vi "Post Destroy.vi"(8 "Error in":errorcluster, 10 "Actor":refnum<class "Actor.lvclass">) -> ()   [LabVIEW 2020, in "jettl.lvlib" / "Actor.lvlib"]
uses:
  Actor.lvlib
  Actor/Actor.lvclass
  Attributes/Attributes/Attributes.lvclass
  Has Destroyed Msg/Has Destroyed Msg.lvlib
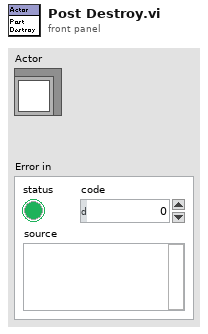
[diagram p1: front panel]
types:
  T1 = typedef "jettl.lvlib/Actor.lvlib/Created Aliases.ctl" = set{string}
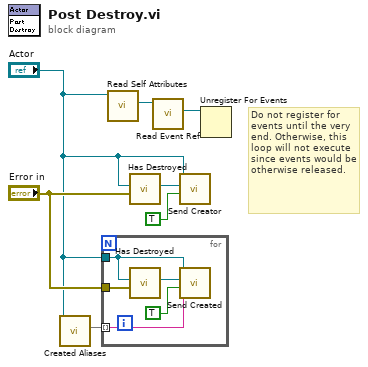
[diagram p0: block diagram]
diagram:
  # "Do not register for events until the very end. Otherwise, this loop will not execute since events would be otherwise released."
  n1 = call-dynamic "Created Aliases.vi"("Actor in"="Actor") -> ("Created Aliases"=w7:T1)  [unwired: 10 in]
  n2 = for {
    tunnel: "Actor" -> [w10]
    tunnel: w7 -> [w12] mode=indexing
    tunnel: "Error in" -> [w8]
    n3 = call "Has Destroyed.vi"("Error"=w8, "Actor"=w10) -> ("Msg"=w9:refnum<class "Msg.lvclass">)  [unwired: 9 in]
    n4 = call-dynamic "Send Created.vi"("Alias"=w12, "Is Priority"=TRUE ("Priority?"), "Msg"=w9, "Actor in"=w10) -> ()  [unwired: 7 in, 1 out]
  }
  n5 = call-dynamic "Read Self Attributes.vi"("Actor in"="Actor") -> ("Self Attributes"=w3:refnum<class "Attributes.lvclass">)  [unwired: 10 in]
  n6 = call "Has Destroyed.vi"("Error"="Error in", "Actor"="Actor") -> ("Msg"=w6:refnum<class "Msg.lvclass">)  [unwired: 9 in]
  n7 = call-dynamic "Read Event Ref.vi"("Attributes in"=w3) -> ("Event Ref"=w2:refnum<event-registration>)  [unwired: 10 in]
  n8 = call-dynamic "Send Creator.vi"("Is Priority"=TRUE ("Priority?"), "Msg"=w6, "Actor in"="Actor") -> ()  [unwired: 8 in, 1 out]
  n9 = Unregister For Events(event registration refnum=w2) -> ()  [unwired: 1 in, 1 out]
